vi "CH_to_Plant_Name.vi"(8 "Error In":errorcluster, 10 "ChannelNo":u8, 11 "Plants_Digital_OP":T1 {"Channel No" items=["7"=7, "11"=11, "12"=12, "13"=13, "15"=15, "16"=16, "18"=18, "29"=29, "32"=32, "33"=33, "35"=35, "36"=36, "37"=37, "38"=38, "40"=40]}) -> (0 "Error Out":errorcluster, 3 "Plant Name":string)   [LabVIEW 2014, in "TimeBasedProd.lvlib"]
uses:
  TypeDef/Plant_OP_Map.ctl
  TypeDef/Plant_OP_Map_CTR.ctl
  ValveCTRL/TypeDef/CHs_List.ctl
  TimeBasedProd.lvlib
  ValveCTRL/ValveCTRL.lvlib
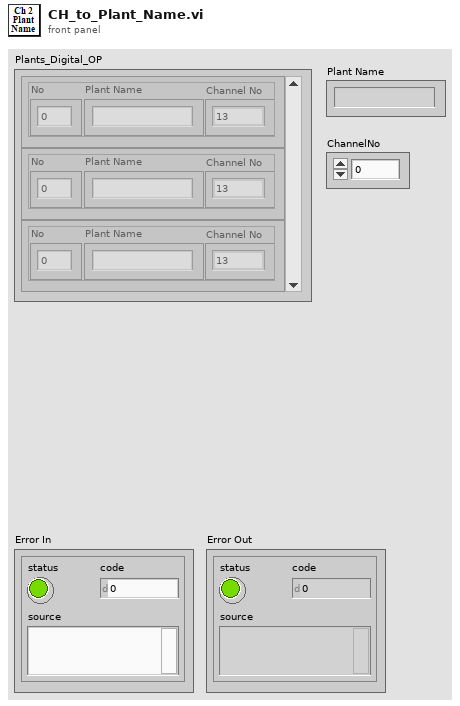
[diagram p1: front panel]
types:
  T1 = typedef "TimeBasedProd.lvlib/Plant_OP_Map.ctl" = T2[]
  T2 = typedef "TimeBasedProd.lvlib/Plant_OP_Map_CTR.ctl" = cluster{"No":u8, "Plant Name":string, "Channel No":T3}
  T3 = typedef "ValveCTRL.lvlib/CHs_List.ctl" = u8
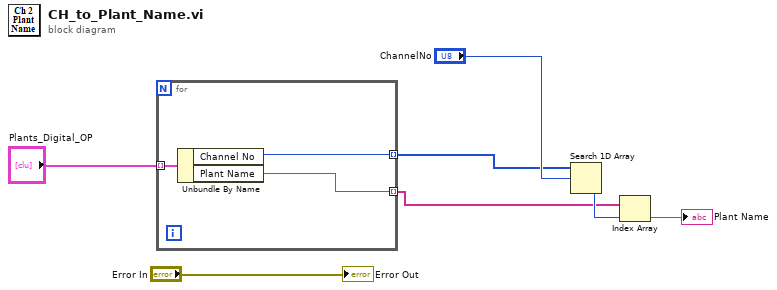
[diagram p0: block diagram]
diagram:
  n1 = for {
    tunnel: "Plants_Digital_OP" -> [w10] mode=indexing
    tunnel: [w9] -> w3 mode=indexing
    tunnel: [w8] -> w2 mode=indexing
    n2 = Unbundle By Name(w10) -> ("Channel No"=w9:T3, "Plant Name"=w8:string)
  }
  n3 = Search 1D Array(1D array=w3, element="ChannelNo") -> (index of element=w5:i32)  [unwired: 1 in]
  n4 = Index Array(array=w2, index=w5) -> (element=→"Plant Name":string)
  "Error Out" <- "Error In"
